vi "DDS update.vi"(8 "error in (no error)":errorcluster, 11 "DDS.lvclass (in)":refnum<class "DDS.lvclass">) -> (0 "error out":errorcluster, 3 "DDS.lvclass":refnum<class "DDS.lvclass">)   [LabVIEW 2015, in "DDS.lvclass"]
uses:
  DDS.lvclass
  DDS.lvclass/DDS.ctl
  Globals.vi
  DDS Library/DDS.lvlib
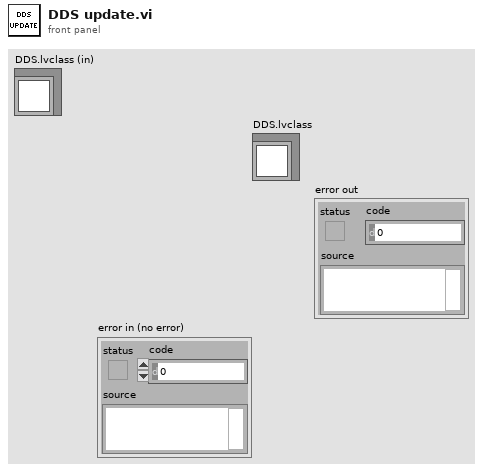
[diagram p1: front panel]
types:
  T1 = typedef "DDS.lvlib/DDS Box Array.ctl" = T2[]
  T2 = typedef "DDS.lvlib/DDS Box Cluster.ctl" = cluster{"DDS box device reference":T3, "Array of DDS Channels (4)":T5, "Enable":bool, "Description":string}
  T3 = typedef "DDS.lvlib/DDS Box Device Reference.ctl" = cluster{"NI USB-8451 device reference":T4, "DIO port":u8, "Serial Clock Rate [kHz]":u16}
  T4 = typedef "ni845xControl.ctl" = refnum<k21>
  T5 = typedef "DDS.lvlib/DDS Channel Array.ctl" = T6[]
  T6 = typedef "DDS.lvlib/DDS Channel.ctl" = cluster{"Power":bool, "Channel Parameters":T7, "RAM Enable":bool, "RAM Dest Type":T8, "RAM Default":cluster{"Frequency [MHz]":dbl, "Amplitude [dBm]":dbl, "Phase Offset [rad]":dbl}, "Array of DDS Profiles (8)":T9, "Description":string}
  T7 = typedef "DDS.lvlib/DDS Channel Parameters.ctl" = cluster{"Ref Clock Rate [MHz]":dbl, "Full Scale Output\nPower [dBm]":dbl}
  T8 = typedef "DDS.lvlib/DDS RAM Destination.ctl" = enum16{"Frequency", "Phase", "Amplitude", "Polar"}
  T9 = typedef "DDS.lvlib/DDS Profile Array.ctl" = T10[]
  T10 = typedef "DDS.lvlib/DDS Profile.ctl" = cluster{"Single Tone":cluster{"Frequency [MHz]":dbl, "Amplitude [dBm]":dbl, "Phase Offset [rad]":dbl}, "RAM Mode ":T11, "Zero-crossing":bool, "No Dwell High":bool, "Function/Static":bool, "RAM Function Settings":string[], "RAM Static Array":dbl[][], "Description":string, "Time Step (us)":T12}
  T11 = typedef "DDS.lvlib/DDS RAM mode.ctl" = enum16{"Direct Switch", "Ramp Up", "Bidirectional Ramp", "Continuous Bidirectional Ramp", "Continuous Recirculate", "Direct Switch 2", "Direct Switch 3", "Direct Switch 4"}
  T12 = typedef "DDS.lvlib/DDS RAM Timestep.ctl" = dbl
  T13 = cluster{"Frequency [MHz]":dbl, "Amplitude [dBm]":dbl, "Phase Offset [rad]":dbl}
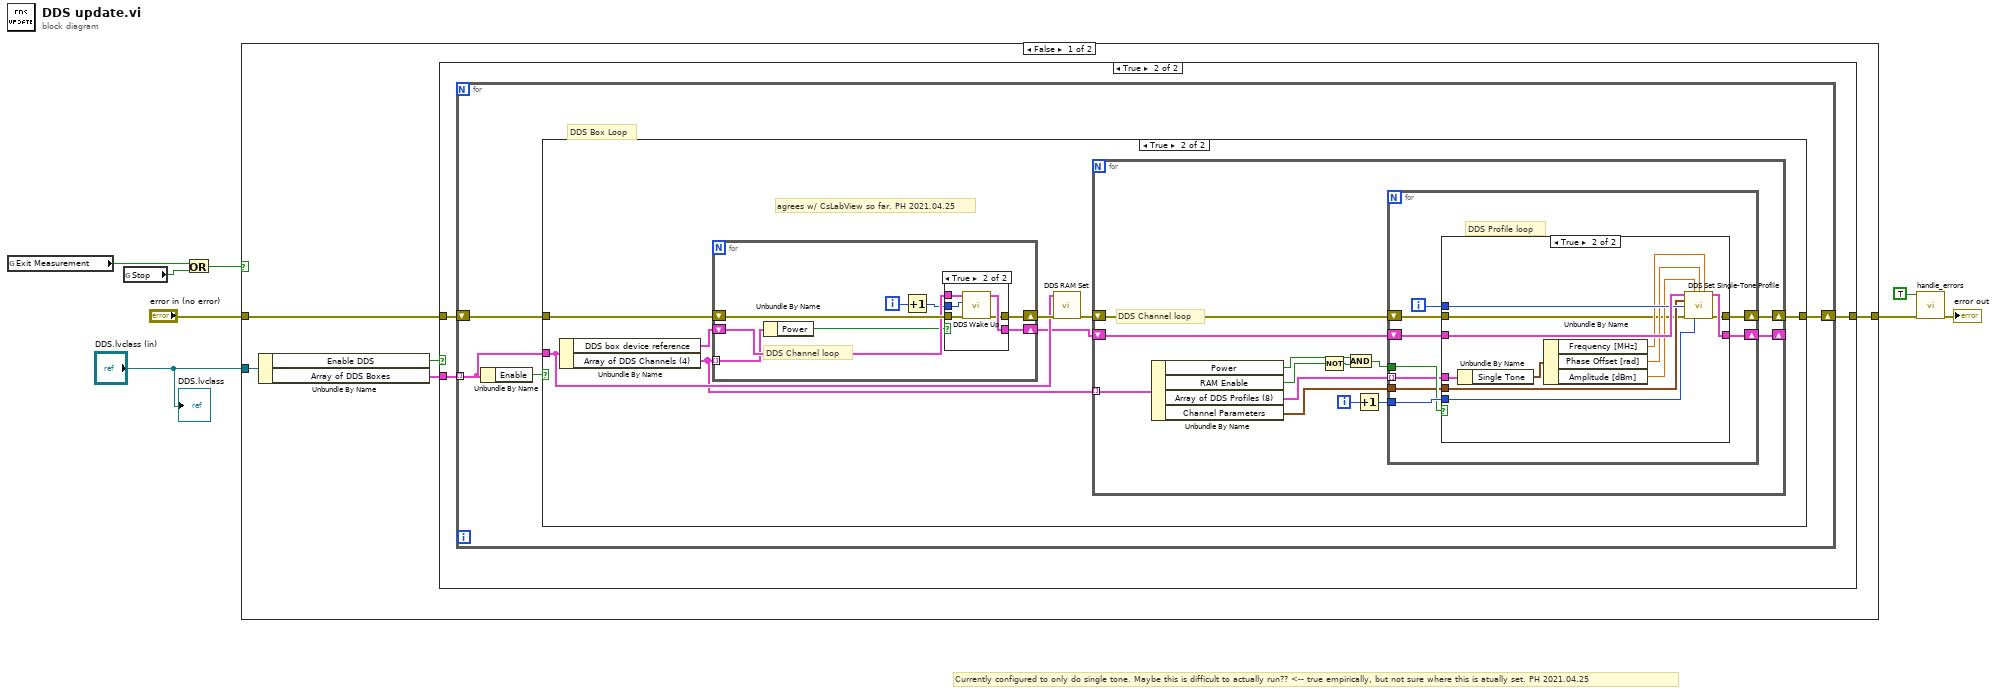
[diagram p0: block diagram]
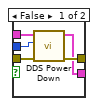
[diagram p5: hidden frame]
diagram:
  # "Currently configured to only do single tone. Maybe this is difficult to actually run?? <-- true empirically, but not sure where this is atually set. PH 2021.04.25"
  n1 = global read "Globals.vi" "Exit Measurement"() -> (w6:bool)
  n2 = global read "Globals.vi" "Stop"() -> (w5:bool)
  n3 = Or(x=w6, y=w5) -> (x .or. y?=w4:bool)
  n4 = case shown="False" w4 {
    tunnel: "error in (no error)" -> [w13 w85]
    tunnel: [w9 w85] -> w2
    tunnel: "DDS.lvclass (in)" -> [w10 _]
    frame False {
      n5 = Unbundle By Name(w10) -> ("Enable DDS"=w12:bool, "Array of DDS Boxes"=w11:T1)
      n6 = case shown="True" w12 {
        tunnel: [w14 w15] -> w9
        tunnel: w13 -> [w14 w17]
        tunnel: w11 -> [_ w16]
        frame False {
        }
        frame True {
          n7 = for {
            shift-right: [w19] -> w15
            shift-left: w17 -> [w18]
            tunnel: w16 -> [w20] mode=indexing
            # "DDS Box Loop"
            n8 = Unbundle By Name(w20) -> ("Enable"=w21:bool)
            n9 = case shown="True" w21 {
              tunnel: w20 -> [_ w27]
              tunnel: w18 -> [w22 w29]
              tunnel: [w22 w24] -> w19
              frame False {
              }
              frame True {
                # "agrees w/ CsLabView so far. PH 2021.04.25"
                n10 = Unbundle By Name(w27) -> ("DDS box device reference"=w30:T3, "Array of DDS Channels (4)"=w25:T5)
                n11 = for {
                  shift-right: [w71] -> w23
                  shift-left: w30 -> [w73]
                  shift-right: [w72] -> w28
                  shift-left: w29 -> [w74]
                  tunnel: w25 -> [w68] mode=indexing
                  i -> [w69]
                  # "DDS Channel loop"
                  n12 = Unbundle By Name(w68) -> ("Power"=w67:bool)
                  n13 = Increment(x=w69) -> (x+1=w70:i32)
                  n14 = case shown="True" w67 {
                    tunnel: w74 -> [w79 w84]
                    tunnel: w73 -> [w78 w83]
                    tunnel: [w77 w80] -> w72
                    tunnel: [w76 w81] -> w71
                    tunnel: w70 -> [w75 w82]
                    frame False {
                      n15 = call "DDS Power Down.vi"("error in (no error)"=w79, "chanel number (1)"=w75, "DDS ref in"=w78) -> ("error out"=w77:errorcluster, "DDS ref out"=w76:T3)  [unwired: 7 in]
                    }
                    frame True {
                      n16 = call "DDS Wake Up.vi"("error in (no error)"=w84, "chanel number (1)"=w82, "DDS ref in"=w83) -> ("error out"=w80:errorcluster, "DDS ref out"=w81:T3)  [unwired: 7 in]
                    }
                  }
                }
                n17 = call "DDS RAM Set.vi"("error in (no error)"=w28, "DDS Box Cluster"=w27) -> ("error out"=w26:errorcluster)  [unwired: 8 in, 1 out]
                n18 = for {
                  shift-right: [w42] -> w24
                  shift-left: w26 -> [w33]
                  shift-right: [w41] -> _
                  shift-left: w23 -> [w43]
                  tunnel: w25 -> [w40] mode=indexing
                  i -> [w38]
                  # "DDS Channel loop"
                  n19 = Unbundle By Name(w40) -> ("Power"=w36:bool, "RAM Enable"=w32:bool, "Array of DDS Profiles (8)"=w39:T9, "Channel Parameters"=w34:T7)
                  n20 = Not(x=w32) -> (.not. x?=w31:bool)
                  n21 = And(x=w36, y=w31) -> (x .and. y?=w35:bool)
                  n22 = Increment(x=w38) -> (x+1=w37:i32)
                  n23 = for {
                    shift-right: [w51] -> w41
                    shift-left: w43 -> [w52]
                    shift-right: [w50] -> w42
                    shift-left: w33 -> [w44]
                    tunnel: w35 -> [w47]
                    tunnel: w37 -> [w49]
                    tunnel: w39 -> [w46] mode=indexing
                    tunnel: w34 -> [w45]
                    i -> [w48]
                    # "DDS Profile loop"
                    n24 = case shown="True" w47 {
                      tunnel: w52 -> [w53 w66]
                      tunnel: w44 -> [w54 w55]
                      tunnel: [w53 w65] -> w51
                      tunnel: [w54 w64] -> w50
                      tunnel: w48 -> [_ w63]
                      tunnel: w49 -> [_ w62]
                      tunnel: w46 -> [_ w61]
                      tunnel: w45 -> [_ w59]
                      frame False {
                        # "If RAM enabled or not powered, \ndo nothing."
                      }
                      frame True {
                        n25 = Unbundle By Name(w61) -> ("Single Tone"=w60:T13)
                        n26 = Unbundle By Name(w60) -> ("Frequency [MHz]"=w58:dbl, "Phase Offset [rad]"=w57:dbl, "Amplitude [dBm]"=w56:dbl)
                        n27 = call "DDS Set Single-Tone Profile.vi"("DDS ref in"=w66, "Amplitude [dBm] (0)"=w56, "Phase Offset [rad] (0)"=w57, "Frequency [MHz] (0)"=w58, "Channel Parameters"=w59, "Profile (0)"=w63, "error in (no error)"=w55, "channel number (1)"=w62) -> ("DDS ref out"=w65:T3, "error out"=w64:errorcluster)  [unwired: 5 in, 1 out]
                      }
                    }
                  }
                }
              }
            }
          }
        }
      }
    }
    frame True {
    }
  }
  n28 = call "handle_errors.vi"("Exit Operation"=TRUE ("Exit Measurement"), "error in (no error)"=w2) -> ("error out"=→"error out":errorcluster)  [unwired: 13 in]
  "DDS.lvclass" <- "DDS.lvclass (in)"
